vi "Read.vi"(8 "error in (no error)":errorcluster, 11 "VISA resource name":refnum<visa-resource-name>) -> (0 "error out":errorcluster, 2 "Measurement":dbl, 3 "VISA resource name out":refnum<visa-resource-name>)   [LabVIEW 2017, in "DmmPwr Simulator.lvlib"]
doc: "Reads and returns a single measurement from the instrument."
uses:
  DmmPwr Simulator.lvlib
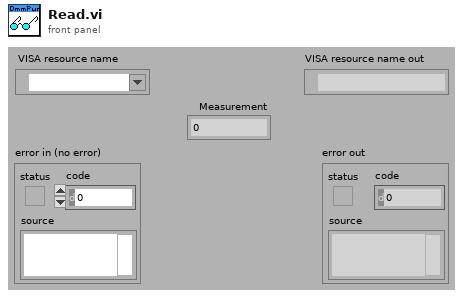
[diagram p1: front panel]
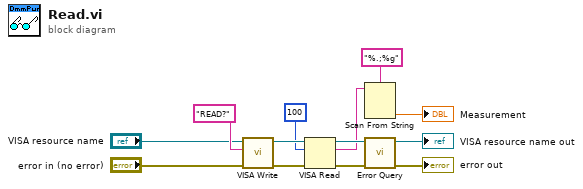
[diagram p0: block diagram]
diagram:
  n1 = call "VISA Write.vi"("error in"="error in (no error)", "write buffer"="READ?", "VISA resource name"="VISA resource name") -> ("error out"=w13:errorcluster, "VISA resource name out"=w12:refnum<visa-resource-name>)  [unwired: 6 in, 1 out]
  n2 = VISA Read(VISA resource name=w12, byte count=u32 100 ("Bytes"), error in (no error)=w13) -> (VISA resource name out=w10:refnum<visa-resource-name>, read buffer=w6:string, error out=w9:errorcluster)  [unwired: 1 out]
  n3 = Scan From String(format string="%.;%g" ("Format String"), input string=w6) -> (output 1=→"Measurement":dbl)  [unwired: 3 in, 3 out]
  n4 = call "Error Query.vi"("error in (no error)"=w9, "VISA resource name"=w10) -> ("error out"=→"error out":errorcluster, "VISA resource name out"=→"VISA resource name out":refnum<visa-resource-name>)  [unwired: 6 in, 2 out]
